vi "Read Measurement (Scope Mode).vi"(8 "error in (no error)":errorcluster, 10 "Measurement Type (11: Measurement Reading 1)":i32(ring)=11 items=["Measurement Reading 1"=11, "Measurement Reading 2"=21, "Measurement Reading 3"=31, "Measurement Reading 4"=41, "Cursor 1 Absolute Amplitude Value"=61, "Cursor Delta V"=62, "Cursor 2 Absolute Amplitude Value"=71, "Cursor Delta T"=72, "Cursor Maximum"=73, "Cursor Average"=74, "Cursor Minimum"=75, "Cursors Frequency"=76], 11 "VISA resource name":refnum<visa-resource-name>) -> (0 "error out":errorcluster, 2 "Measurement Value":dbl format="%#.3e", 3 "VISA resource name out":refnum<visa-resource-name>)   [LabVIEW 2014, in "Fluke 190 Series II.lvlib"]
doc: "Queries the measurement result from the Scopemeter in scope mode."
uses:
  Fluke 190 Series II.lvlib
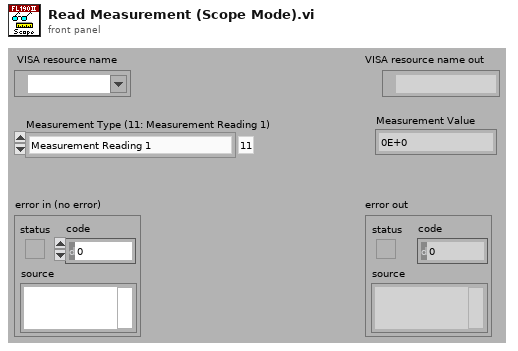
[diagram p1: front panel]
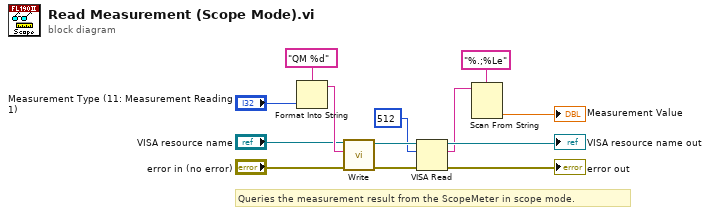
[diagram p0: block diagram]
diagram:
  # "Queries the measurement result from the ScopeMeter in scope mode."
  n1 = Format Into String(format string="QM %d", "Measurement Type (11: Measurement Reading 1)") -> (resulting string=w11:string)  [unwired: 2 in, 1 out]
  n2 = call "Write.vi"("error in (no error)"="error in (no error)", "Write Buffer"=w11, "VISA resource name"="VISA resource name") -> ("error out"=w7:errorcluster, "VISA resource name out"=w8:refnum<visa-resource-name>)  [unwired: 7 out]
  n3 = VISA Read(VISA resource name=w8, byte count=u32 512, error in (no error)=w7) -> (VISA resource name out=→"VISA resource name out":refnum<visa-resource-name>, read buffer=w4:string, error out=→"error out":errorcluster)  [unwired: 1 out]
  n4 = Scan From String(format string="%.;%Le", input string=w4) -> (output 1=→"Measurement Value":dbl)  [unwired: 2 in, 4 out]
